vi "set socket option.vi"(7 "level":i32, 8 "error in":errorcluster, 9 "option value":string, 10 "option":i32, 11 "socket":i32) -> (0 "error out":errorcluster)   [LabVIEW 2013, in "lvnano.lvlib"]
doc: "NN_EXPORT int nn_setsockopt (int s, int level, int option, const void *optval,\n size_t optvallen);"
uses:
  lvnano.lvlib
  get last error code.vi
  get error string from code.vi
  <vilib>/Utility/error.llb/Error Cluster From Error Code.vi
  lvnanomsg.dll
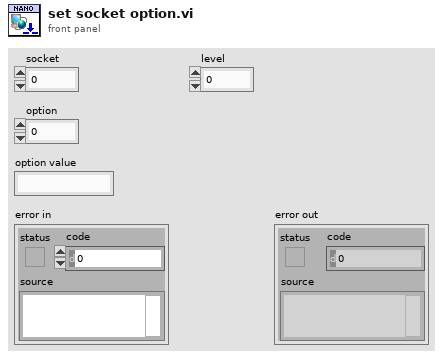
[diagram p1: front panel]
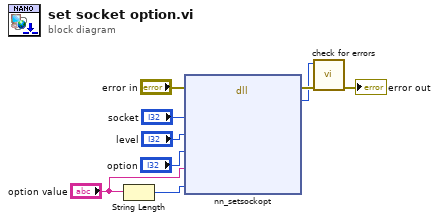
[diagram p0: block diagram]
diagram:
  n1 = String Length(string="option value") -> (length=w2:i32)
  n2 = dll-call lib="C:/Users/Daniel/Documents/nanomsg/lvnano/lvnanomsg.*" fn="nn_setsockopt"(error in="error in", "socket"="socket", "level"="level", "option"="option", "option value"="option value", "option length"=w2) -> (error out=w5:errorcluster, "error"=w1:i32)  [unwired: 7 in, 1 out]
  n3 = call "check for errors.vi"("error in"=w5, "function return"=w1) -> ("error out"=→"error out":errorcluster)  [unwired: 9 in]
